vi "Experiment-3_4526.vi"() -> ()   [LabVIEW 2021]
panel:
  out "data":dynamicdata(graph)
  in  "error in":errorcluster
  in  "device name":tag="Experiment-3_4526"
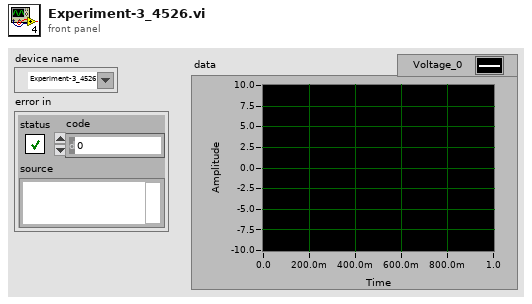
[diagram p1: front panel]
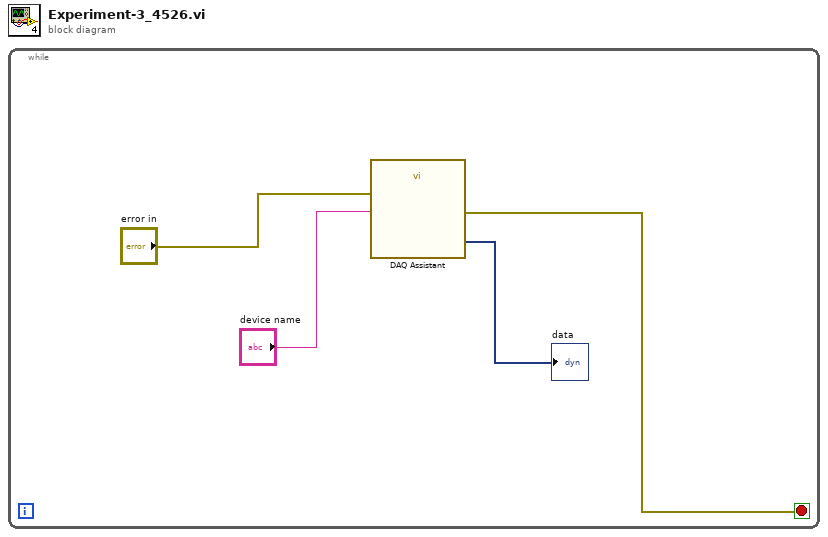
[diagram p0: block diagram]
diagram:
  n1 = while {
    stop <- w1 stop-if-true
    n2 = call "DAQ Assistant"("error in"="error in", "device name"="device name") -> ("data"=→"data":dynamicdata, "error out"=w1:errorcluster)  [unwired: 15 in, 1 out]
  }
